vi "Set uWave Switch.vi"(0 "uWave Switch":i32(listbox)) -> ()   [LabVIEW 2010]
uses:
  MWC Global.vi
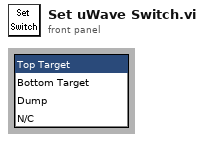
[diagram p1: front panel]
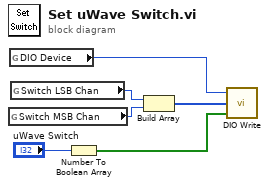
[diagram p0: block diagram]
diagram:
  n1 = global read "MWC Global.vi" "Switch MSB Chan"() -> (w5:i32)
  n2 = global read "MWC Global.vi" "DIO Device"() -> (w3:i32)
  n3 = global read "MWC Global.vi" "Switch LSB Chan"() -> (w4:i32)
  n4 = Number To Boolean Array(number="uWave Switch") -> (Boolean array=w1:bool[])
  n5 = Build Array(w4, w5) -> (w2:i32[])
  n6 = call "DIO Write.vi"("Data"=w1, "Channels"=w2, "device"=w3) -> ()  [unwired: 1 out]
